vi "Send Block Location (SubVI).vi"(0 "Bounding Box":u64, 7 "Data Valid":bool, 11 "EOI Out":bool) -> ()   [LabVIEW 2015]
uses:
  <vilib>/rvi/interface/RandomDataEmulation/niFpgaRandomDataHandleErrors.vi
  <vilib>/rvi/DataTransferAndStorage/Container/XNode/niFpgaContainer.xnode
  <vilib>/rvi/interface/RandomDataEmulation/nirviRandomDataFpgaReadWriteTemplate.vi
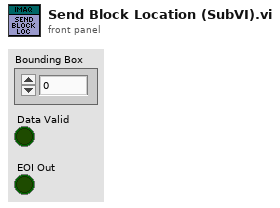
[diagram p1: front panel]
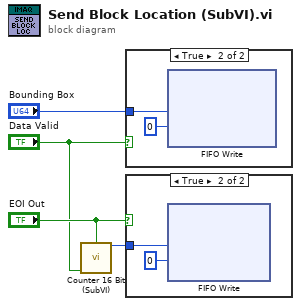
[diagram p0: block diagram]
diagram:
  n1 = call "Counter 16 Bit (SubVI).vi"("RESET"="EOI Out", "Enable"="Data Valid") -> ("Count"=w2:u16)  [unwired: 11 in, 2 out]
  n2 = case shown="True" "Data Valid" {
    tunnel: "Bounding Box" -> [_ w5]
    frame False {
    }
    frame True {
      n3 = xnode ("FIFO Write")("Element"=w5, "Timeout"=0) -> ()  [unwired: 1 in, 2 out]
    }
  }
  n4 = case shown="True" "EOI Out" {
    tunnel: w2 -> [_ w7]
    frame False {
    }
    frame True {
      n5 = xnode ("FIFO Write")("Element"=w7, "Timeout"=0) -> ()  [unwired: 1 in, 2 out]
    }
  }
